vi "2D Array Reorder.vi"(0 "2D Array Data witjh Header":string[][](array[string]), 5 "Header Order":string[](array[string]), 11 "error in (no error)":errorcluster) -> (4 "Reordered Data without Header":string[][](array[string]), 15 "error out":errorcluster)   [LabVIEW 2023, in "Utilities.lvlib"]
uses:
  Utilities.lvlib
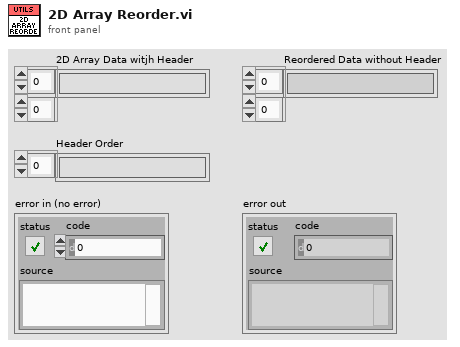
[diagram p1: front panel]
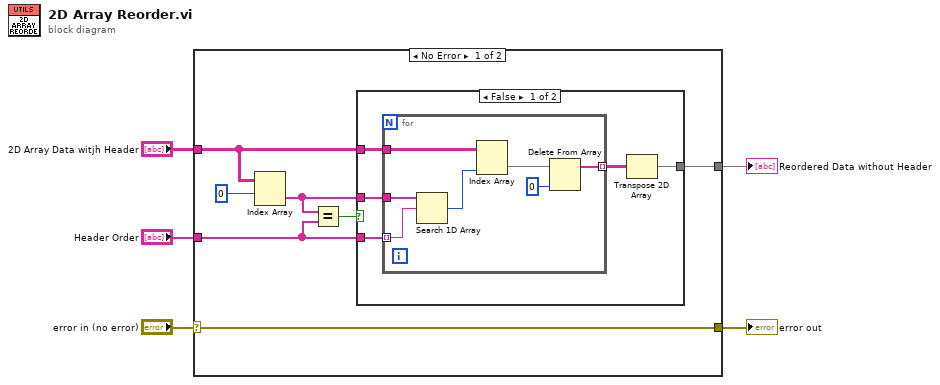
[diagram p0: block diagram]
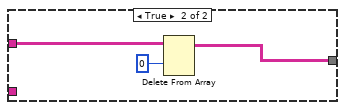
[diagram p2: hidden frame]
diagram:
  n1 = case shown="No Error" "error in (no error)" {
    selector: "error in (no error)" -> [w6 w28]
    tunnel: "2D Array Data witjh Header" -> [w11 w29]
    tunnel: [w10 w29] -> w4
    tunnel: "Header Order" -> [w8 _]
    tunnel: [w6 w28] -> w1
    frame No Error {
      n2 = Index Array(array=w11, index (row)=0) -> (element=w9:string[])  [unwired: 1 in]
      n3 = Equal?(x=w9, y=w8) -> (x = y?=w7:bool)
      n4 = case shown="False" w7 {
        tunnel: w11 -> [w17 w27]
        tunnel: [w15 w26] -> w10
        tunnel: w9 -> [w14 _]
        tunnel: w8 -> [w13 _]
        frame False {
          n5 = for {
            tunnel: w13 -> [w23] mode=indexing
            tunnel: w14 -> [w24]
            tunnel: w17 -> [w22]
            tunnel: [w18] -> w16 mode=indexing
            n6 = Search 1D Array(1D array=w24, element=w23) -> (index of element=w21:i32)  [unwired: 1 in]
            n7 = Index Array(array=w22, index (col)=w21) -> (element=w20:string[])  [unwired: 1 in]
            n8 = Delete From Array(array=w20, index=0) -> (array with subset deleted=w18:string[])  [unwired: 1 in, 1 out]
          }
          n9 = Transpose 2D Array(2D array=w16) -> (transposed array=w15:string[][])
        }
        frame True {
          n10 = Delete From Array(array=w27, index (row)=0) -> (array with subset deleted=w26:string[][])  [unwired: 2 in, 1 out]
        }
      }
    }
    frame Error {
    }
  }
  "error out" <- w1
  "Reordered Data without Header" <- w4
